vi "Do.vi"(8 "error in (no error)":errorcluster, 10 "Actor in":refnum<class "Actor.lvclass">, 11 "Set Ratios Msg":refnum<class "Set Ratios Msg.lvclass">) -> (0 "error out":errorcluster, 2 "Actor out":refnum<class "Actor.lvclass">)   [LabVIEW 2017, in "BNT_DAQmx.lvlib" / "Set Ratios Msg.lvclass"]
doc: "This VI delivers the message to the actor by calling the appropriate method(s) on the actor."
uses:
  Set Ratios Msg.lvclass
  <vilib>/ActorFramework/Actor/Actor.lvclass
  C:/User/Brand/LVP/Acc/VacuumHeating/Packages/CSPP_Core/Messages/CSPP_PVUpdate Msg/CSPP_PVUpdate Msg.lvclass
  BNT_DAQmx-MCSV-DOPWM/BNT_DAQmx-MCSV-DOPWM.lvclass
  C:/Program Files (x86)/National Instruments/LabVIEW 2017/vi.lib/ActorFramework/Actor/Actor.lvclass
  CSPP_Core/Messages/CSPP_PVUpdate Msg/CSPP_PVUpdate Msg.lvclass/CSPP_PVUpdate Msg.ctl
  CSPP_Core/Classes/CSPP_ProcessVariables/ProcessVariable/PV.lvclass/PV.ctl
  Set Ratios Msg.lvclass/Set Ratios Msg.ctl
  CSPP_Core/Classes/CSPP_ProcessVariables/ProcessVariable/PV.lvclass
  CSPP_Core/Messages/CSPP_PVUpdate Msg/CSPP_PVUpdate Msg.lvclass
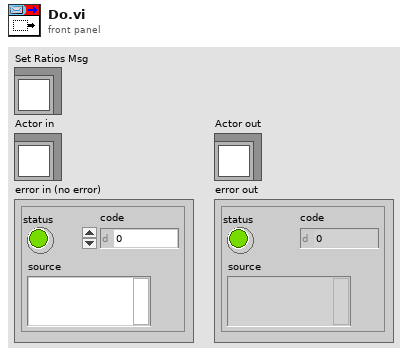
[diagram p1: front panel]
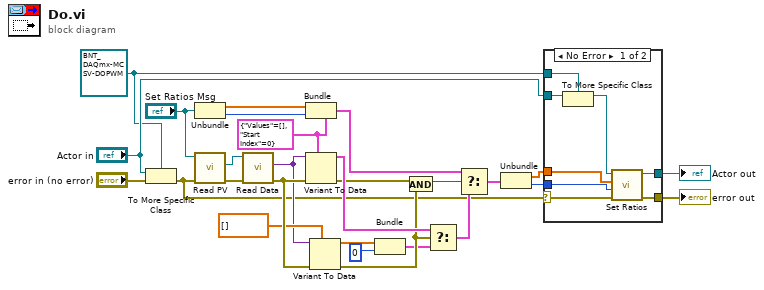
[diagram p0: block diagram]
diagram:
  w7 = cluster{"Values":dbl[], "Start Index":i32} {"Values"=[], "Start Index"=0} ("Type")
  w23 = refnum<class "BNT_DAQmx-MCSV-DOPWM.lvclass"> refnum ("Actor in")
  n1 = To More Specific Class(target class=w23, reference="Actor in", error in="error in (no error)") -> (error out=w3:errorcluster)  [unwired: 1 out]
  n2 = Unbundle ("Pre-Unbundler")("Set Ratios Msg") -> (w9:dbl[], w10:i32)
  n3 = call "Read PV.vi"("error in (no error)"=w3, "CS++PVUpdate Msg in"="Set Ratios Msg") -> ("error out"=w5:errorcluster, "PV"=w8:refnum<class "PV.lvclass">)  [unwired: 7 in, 1 out]
  n4 = call "Read Data.vi"("error in (no error)"=w5, "PV in"=w8) -> ("error out"=w13:errorcluster, "Data"=w11:variant)  [unwired: 7 in, 1 out]
  n5 = Bundle ("Pre-Bundler")(cluster=w7, "Values"=w9, "Start Index"=w10) -> (w6:cluster{"Values":dbl[], "Start Index":i32})
  n6 = Variant To Data(error in=w13, type=w7, Variant=w11) -> (data=w19:cluster{"Values":dbl[], "Start Index":i32}, error out=w2:errorcluster)
  n7 = Variant To Data(error in=w13, type=dbl[] [] ("Values"), Variant=w11) -> (data=w14:dbl[], error out=w18:errorcluster)
  n8 = Bundle ("Pre-Bundler")("Values"=w14, "Start Index"=0) -> (w16:cluster{"Values":dbl[], "Start Index":i32})  [unwired: 1 in]
  n9 = And(x=w2, y=w18) -> (x .and. y?=w17:bool)
  n10 = Select ("MainSelect")(t=w19, s=w18, f=w16) -> (s? t:f=w20:cluster{"Values":dbl[], "Start Index":i32})
  n11 = Select ("MainSelect")(t=w6, s=w17, f=w20) -> (s? t:f=w1:cluster{"Values":dbl[], "Start Index":i32})
  n12 = Unbundle ("Main-Unbundler")(w1) -> ("Values"=w22:dbl[], "Start Index"=w21:i32)
  n13 = case shown="No Error" w3 {
    selector: w3 -> [w33 w37]
    tunnel: [w35 w37] -> w26
    tunnel: [w34 w36] -> w25
    tunnel: "Actor in" -> [w32 w36]
    tunnel: w23 -> [w31 _]
    tunnel: w22 -> [w29 _]
    tunnel: w21 -> [w28 _]
    frame No Error {
      n14 = To More Specific Class(target class=w31, reference=w32) -> (specific class reference=w30:refnum<class "BNT_DAQmx-MCSV-DOPWM.lvclass">)  [unwired: 1 in, 1 out]
      n15 = call "Set Ratios.vi"("error in"=w33, "Start Index"=w28, "PWM Ratios"=w29, "BNT_DAQmx-MCSV-DOPWM in"=w30) -> ("error out"=w35:errorcluster, "BNT_DAQmx-MCSV-DOPWM out"=w34:refnum<class "BNT_DAQmx-MCSV-DOPWM.lvclass">)  [unwired: 6 in]
    }
    frame Error {
    }
  }
  "error out" <- w26
  "Actor out" <- w25
